vi "Appearance Page.vi"() -> ()   [LabVIEW 2017, in "2D Plot.lvclass"]
uses:
  <vilib>/Math Plots/2D Math Plots/2D Plot/2D Plot/2D Plot.lvclass
  <vilib>/Math Plots/2D Math Plots/2D Plot/2D Plot/Typedef/Graph General Property.ctl
  <vilib>/Math Plots/2D Math Plots/2D Plot/Action String/2DMathPlot Ctrl Act Queue.ctl
  <vilib>/Math Plots/2D Math Plots/2D Plot/Action String/2DMathPlot Ctrl Act Cluster.ctl
  <vilib>/Math Plots/2D Math Plots/2D Plot/Action String/2DMathPlot State Class.ctl
  <vilib>/Math Plots/2D Math Plots/2D Plot/2D Plot/Typedef/Dialog State.ctl
  <vilib>/Math Plots/2D Math Plots/2D Plot/2D Plot/Typedef/Temp Graph Property Action.ctl
  <vilib>/Math Plots/2D Math Plots/2D Plot/2D Plot/Typedef/Temp Graph State.ctl
panel:
  in  "Event Registration":refnum<event-registration>
  in  "Control Ref Queue":T1
  out "Graph General Out":T2
  in  "Graph General In":T2
  in  "Legend:Plots Shown":u32=1 caption="Plots shown" min=1
  in  "Autosize Legend":bool caption="Auto size to plot names"
  in  "Cursor Palette Visible":bool caption="Show cursor legend"
  in  "Legend:Visible":bool caption="Show plot legend"
  in  "Scale Legend:Visible":bool caption="Show scale legend"
  in  "Palette:Visible":bool caption="Show graph palette"
  in  "X Scrollbar Visible":bool caption="Show x scroll bar"
  in  "Height":u32 step=1
  in  "Width":u32 step=1
  in  "Enabled State":T3(radio)
  in  "Caption.Visible":bool caption="Caption"
  in  "Caption.Text":string caption="Caption Text"
  in  "Label.Text":string caption="Label Text"
  in  "Label.Visible":bool caption="Label"
  # "Caption"
  # "Label"
  # "Enabled State"
  # "Size"
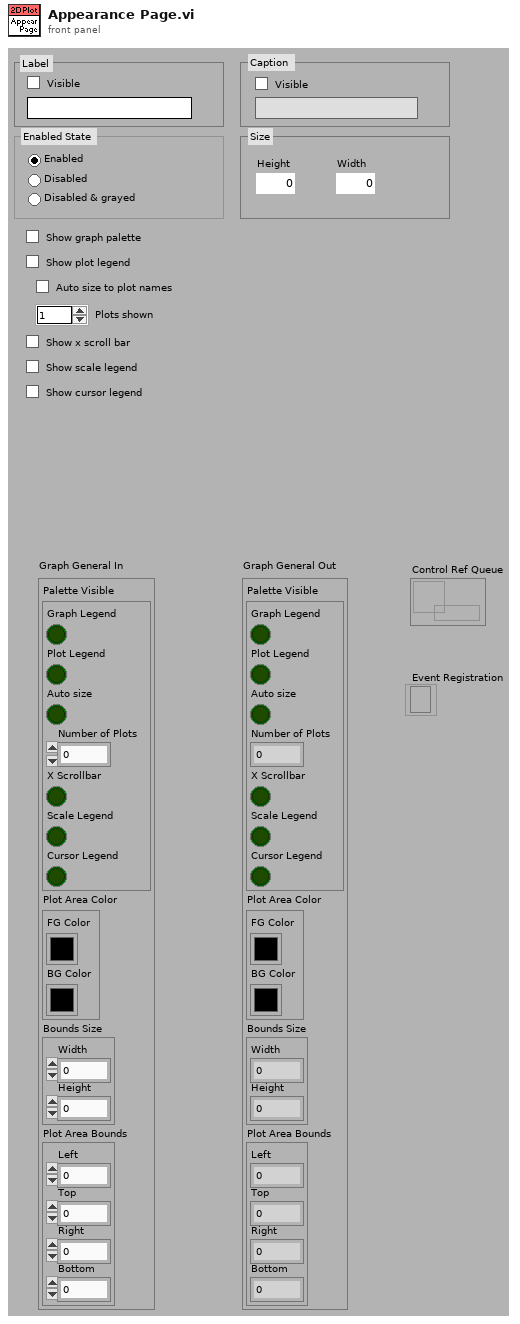
[diagram p1: front panel]
types:
  T1 = typedef "2DMathPlot Ctrl Act Queue.ctl" = refnum<queue>
  T2 = typedef "2D Plot.lvclass/Graph General Property.ctl" = cluster{"Palette Visible":cluster{"Graph Legend":bool, "Plot Legend":bool, "Auto size":bool, "Number of Plots":u32, "X Scrollbar":bool, "Scale Legend":bool, "Cursor Legend":bool}, "Plot Area Color":cluster{"FG Color":u32, "BG Color":u32}, "Bounds Size":cluster{"Width":u32, "Height":u32}, "Plot Area Bounds":cluster{"Left":i16, "Top":i16, "Right":i16, "Bottom":i16}}
  T3 = enum32{"Enabled", "Disabled", "Disabled & grayed", "Multiple Values"}
  T4 = typedef "2D Plot.lvclass/Dialog State.ctl" = enum16{"Initialize", "Read Property", "Write Property", "Idle", "Exit"}
  T5 = typedef "2DMathPlot Ctrl Act Cluster.ctl" = cluster{"Plot Area Ref":refnum<vi>, "Z Axis Ref":refnum<vi>, "Legend Ref":refnum<vi>, "XControl Ref":refnum<vi>, "Facade Ref":refnum<vi>, "Display State Change Class":T6}
  T6 = typedef "2DMathPlot State Class.ctl" = enum16{"Update All (Undo)", "Update General", "Update Appearance", "Update Format", "Update Scale", "Update Marker", "Update Cursor", "None"}
  T7 = typedef "2D Plot.lvclass/Temp Graph State.ctl" = enum16{"Create", "Update Graph", "Update Property Only", "Get Plot Name", "Get Axis Name", "Destory"}
  T8 = typedef "2D Plot.lvclass/Temp Graph Property Action.ctl" = enum16{"Appearance Property", "Format Property", "Plots Property", "Scales Property"}
  T9 = cluster{"Left":i16, "Top":i16, "Right":i16, "Bottom":i16}
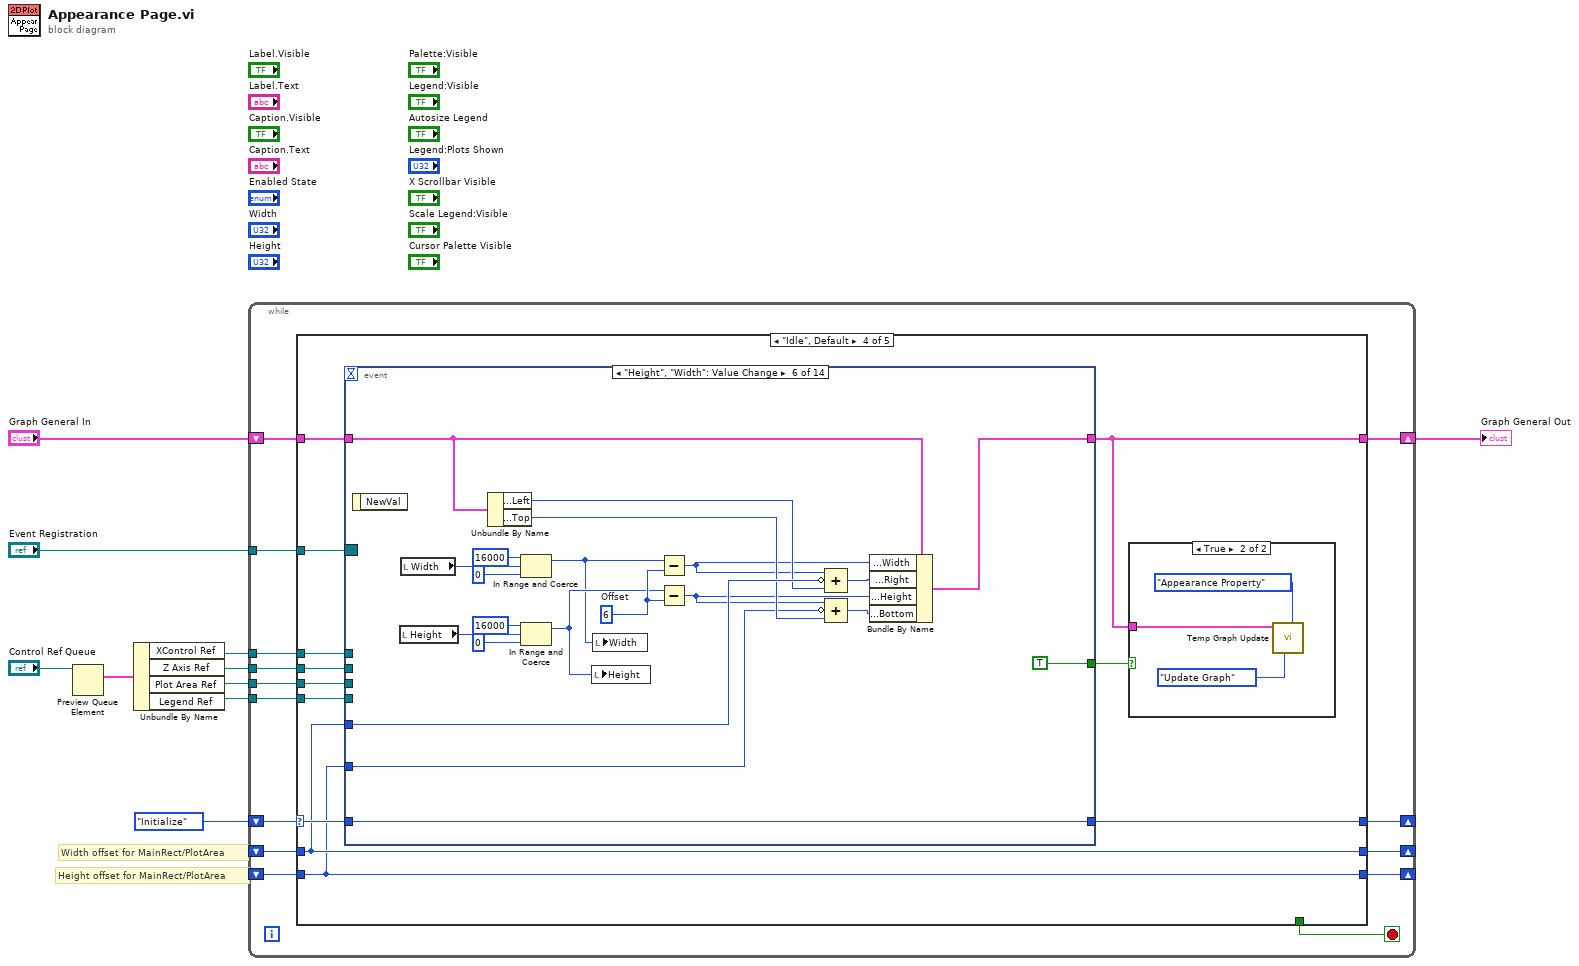
[diagram p0: block diagram]
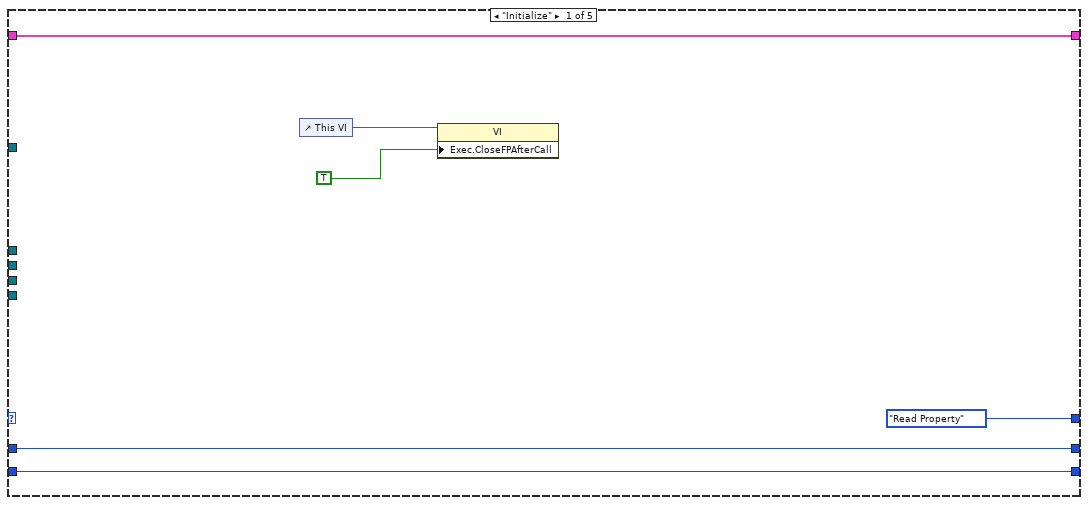
[diagram p2: hidden frame]
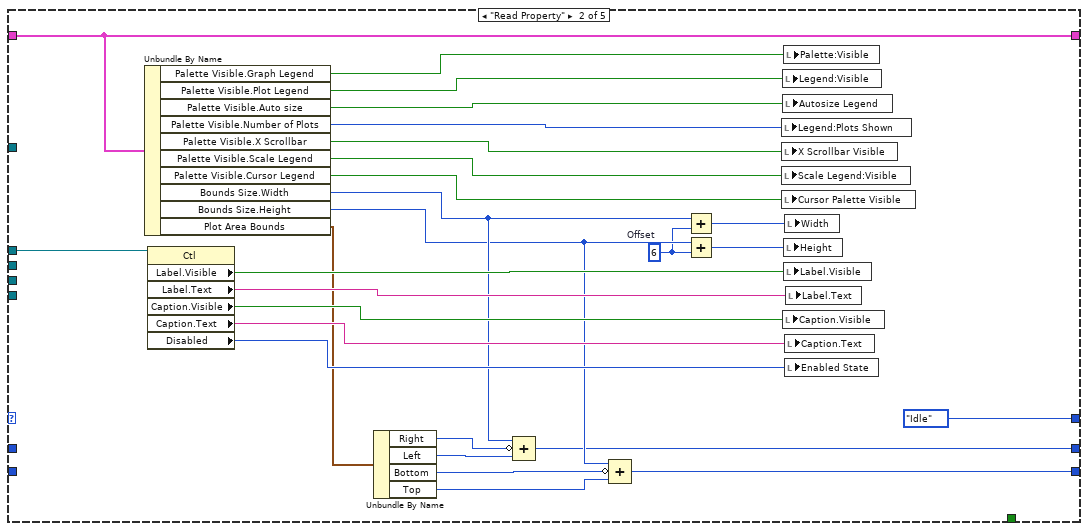
[diagram p3: hidden frame]
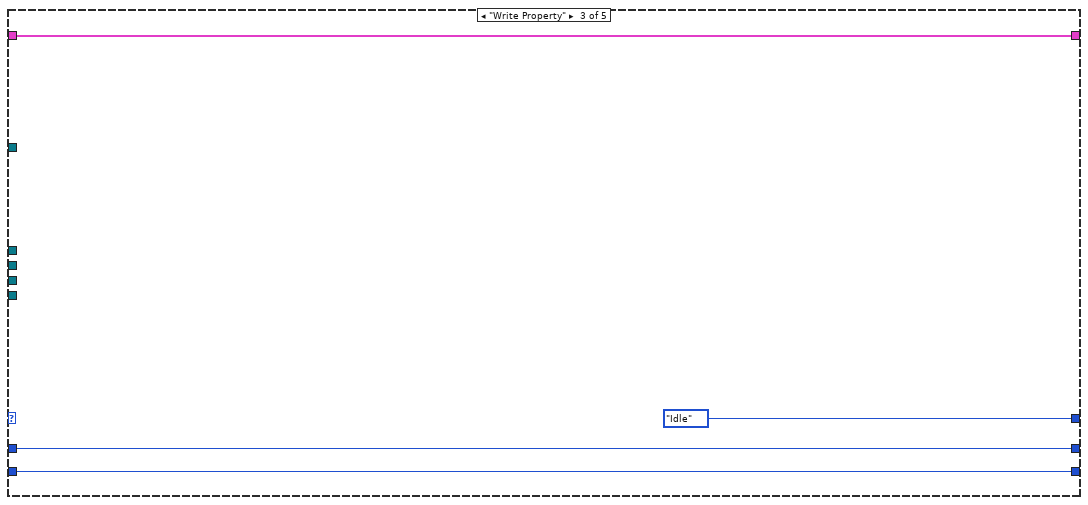
[diagram p4: hidden frame]
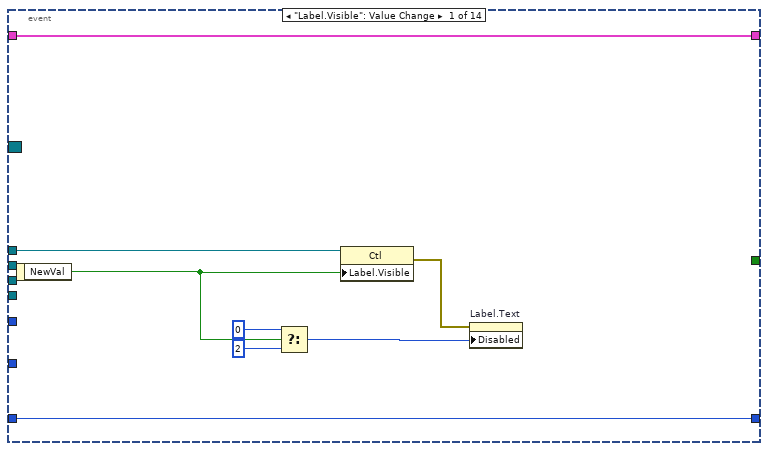
[diagram p6: hidden frame]
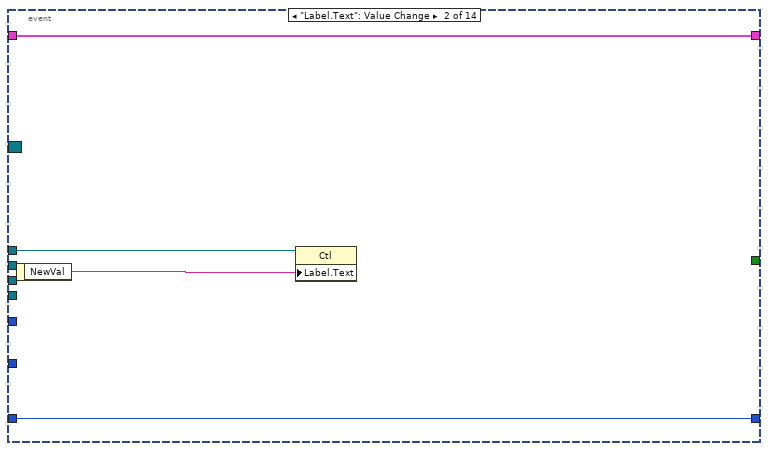
[diagram p7: hidden frame]
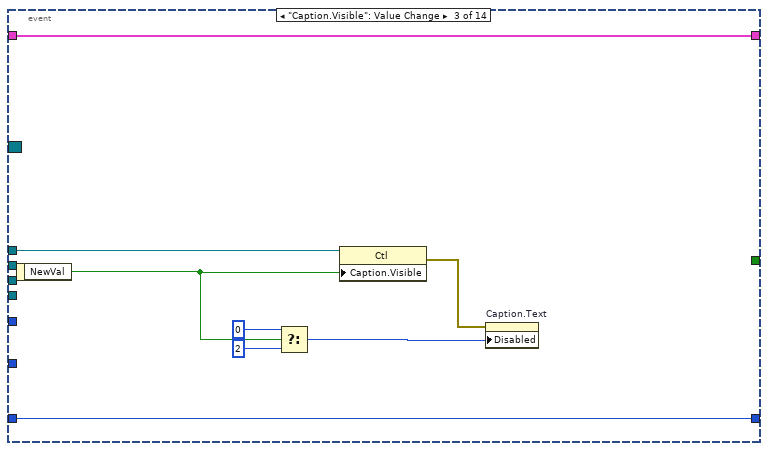
[diagram p8: hidden frame]
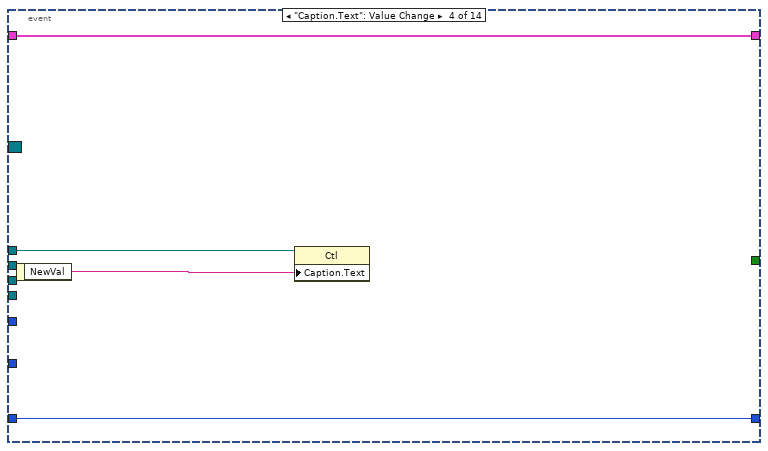
[diagram p9: hidden frame]
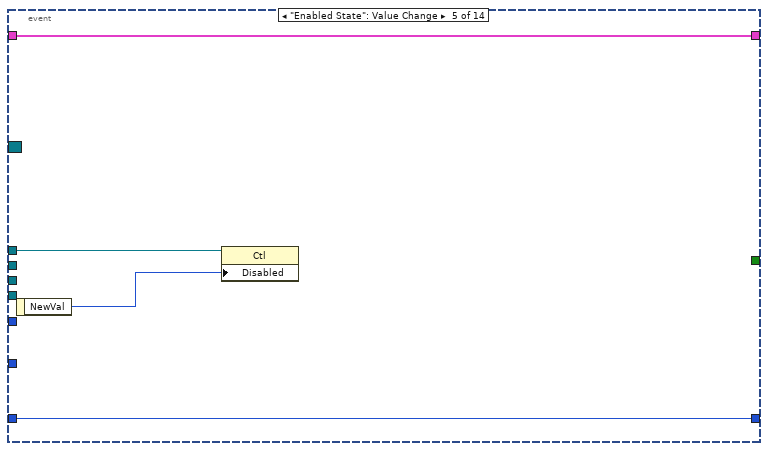
[diagram p10: hidden frame]
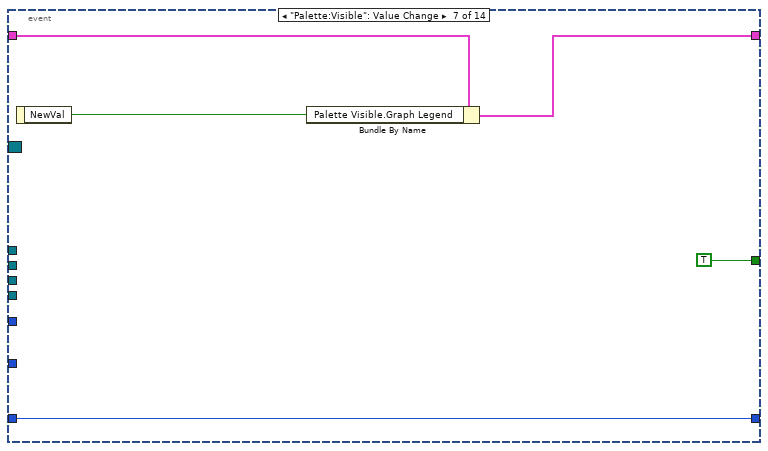
[diagram p11: hidden frame]
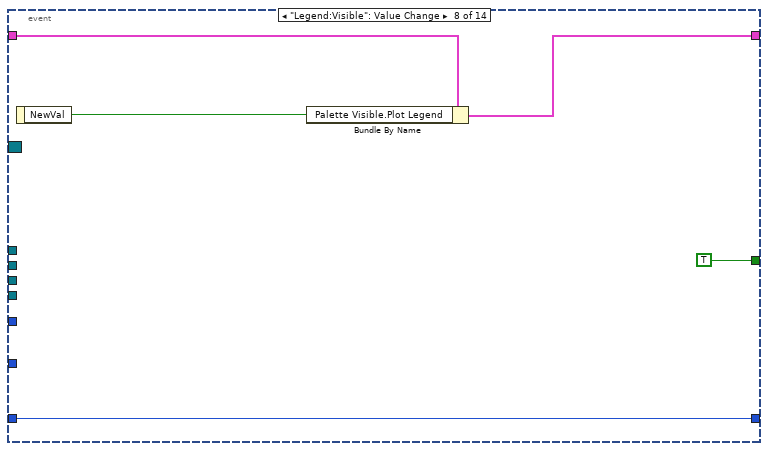
[diagram p12: hidden frame]
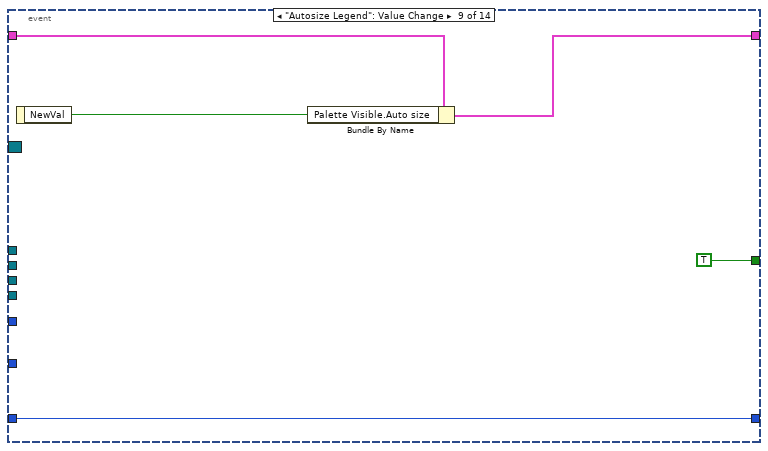
[diagram p13: hidden frame]
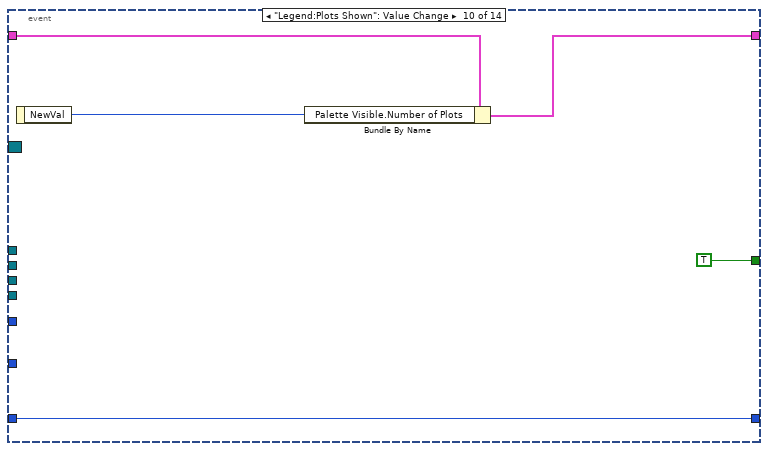
[diagram p14: hidden frame]
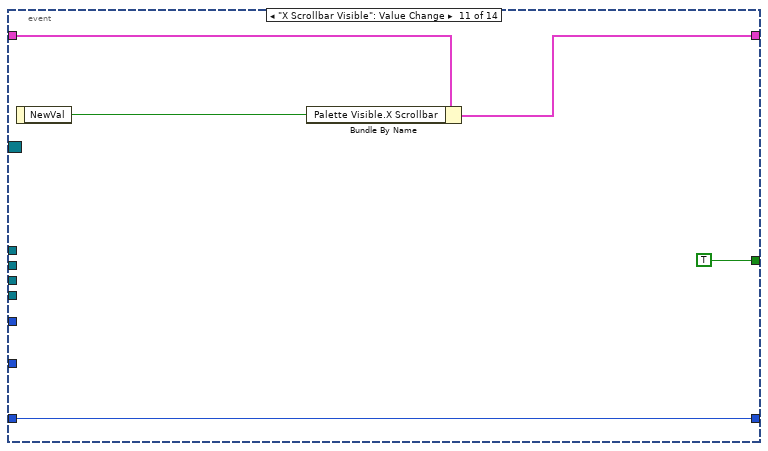
[diagram p15: hidden frame]
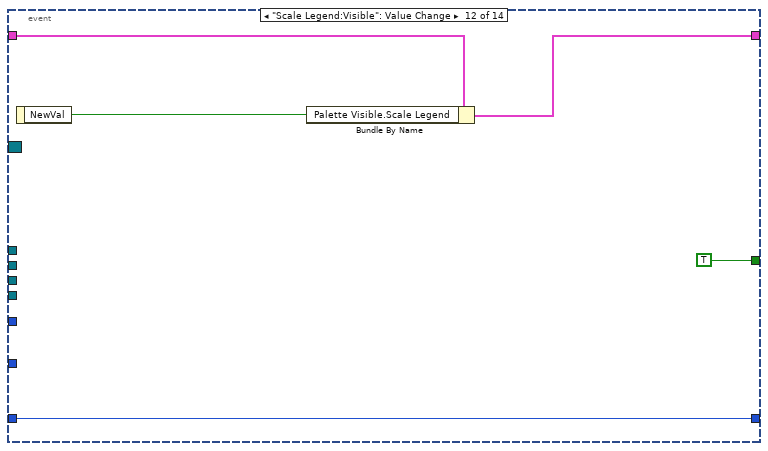
[diagram p16: hidden frame]
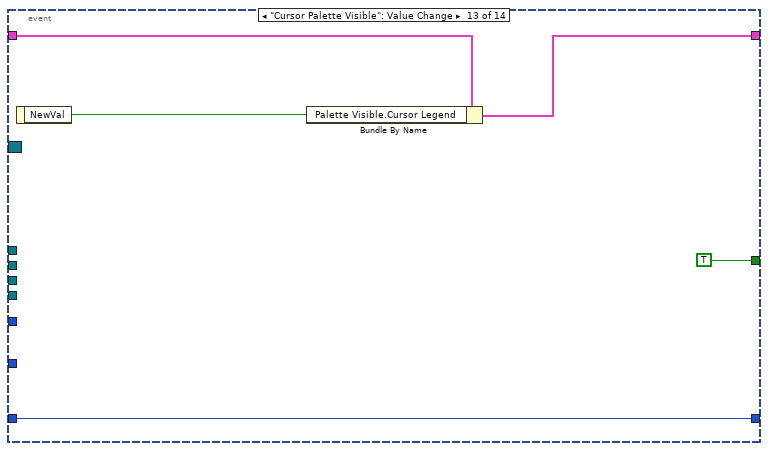
[diagram p17: hidden frame]
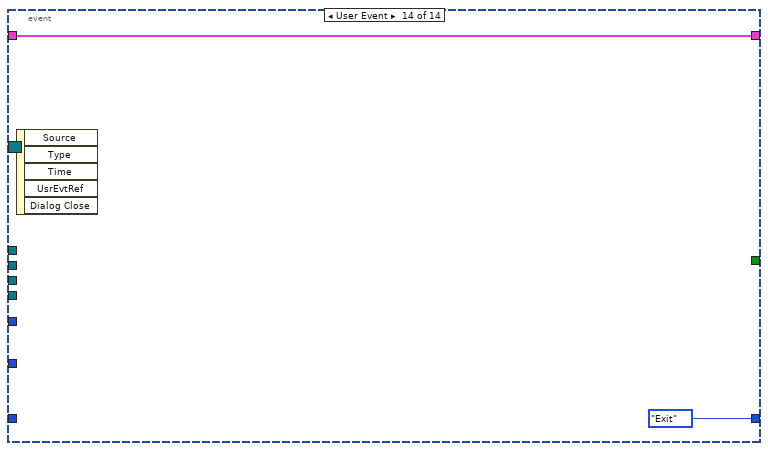
[diagram p18: hidden frame]
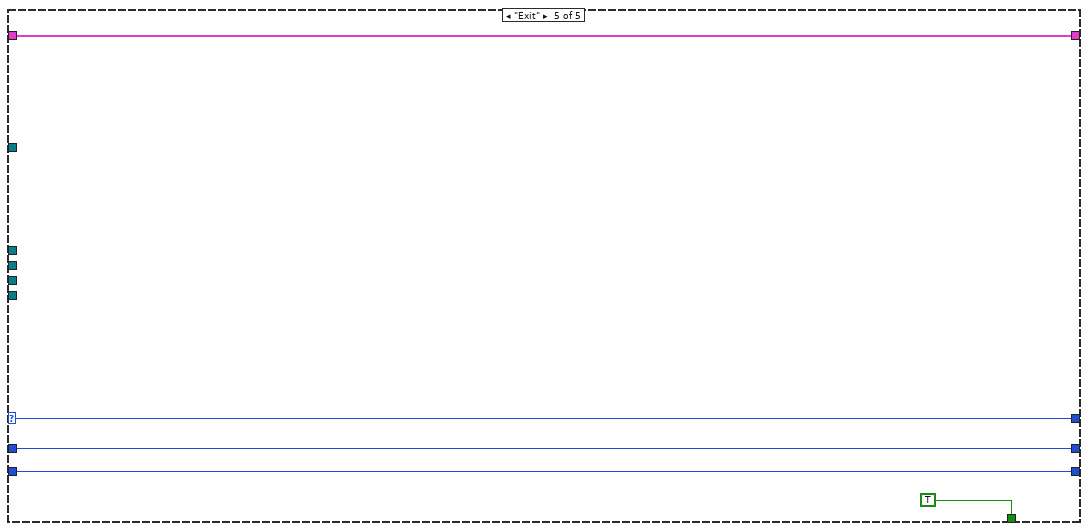
[diagram p19: hidden frame]
diagram:
  # "Height offset for MainRect/PlotArea"
  # "Width offset for MainRect/PlotArea"
  n1 = Preview Queue Element(queue="Control Ref Queue") -> (element=w2:T5)  [unwired: 1 in, 4 out]
  n2 = Unbundle By Name(w2) -> ("XControl Ref"=w6:refnum<vi>, "Z Axis Ref"=w5:refnum<vi>, "Plot Area Ref"=w4:refnum<vi>, "Legend Ref"=w1:refnum<vi>)
  n3 = while {
    shift-right: [w22] -> _
    shift-left: Dialog_State."Initialize" ("Enum") -> [w24]
    shift-right: [w21] -> w9
    shift-left: "Graph General In" -> [w20]
    tunnel: w6 -> [w19]
    tunnel: w5 -> [w18]
    tunnel: w4 -> [w17]
    tunnel: "Event Registration" -> [w16]
    shift-right: [w15] -> _
    shift-left: _ -> [w13]
    shift-right: [w14] -> _
    shift-left: _ -> [w12]
    tunnel: w1 -> [w11]
    stop <- w23 stop-if-true
    n4 = case shown="\"Idle\", Default" w24 {
      selector: w24 -> [_ _ _ w67 w166]
      tunnel: [_ _ _ _ TRUE] -> w23
      tunnel: [Dialog_State."Read Property" ("Enum") Dialog_State."Idle" ("Enum") Dialog_State."Idle" ("Enum") w68 w166] -> w22
      tunnel: [w27 w43 w60 w62 w165] -> w21
      tunnel: w20 -> [w27 w43 w60 w73 w165]
      tunnel: w19 -> [_ w49 _ w72 _]
      tunnel: w18 -> [_ _ _ w71 _]
      tunnel: w17 -> [_ _ _ w70 _]
      tunnel: w16 -> [_ _ _ w69 _]
      tunnel: [w26 w34 w59 w65 w164] -> w15
      tunnel: [w25 w35 w58 w64 w163] -> w14
      tunnel: w13 -> [w26 _ w59 w65 w164]
      tunnel: w12 -> [w25 _ w58 w64 w163]
      tunnel: w11 -> [_ _ _ w63 _]
      frame "Initialize" {
        n5 = control-ref of="This VI"() -> (w29:refnum<vi>)
        n6 = property class="VI"(reference=w29, "Exec.CloseFPAfterCall"=TRUE ("Execution:Close After Call")) -> ()  [unwired: 1 in, 2 out]
      }
      frame "Read Property" {
        w31 = u32 6  # Offset
        n7 = Unbundle By Name(w43) -> ("Palette Visible.Graph Legend"=w56:bool, "Palette Visible.Plot Legend"=w55:bool, "Palette Visible.Auto size"=w54:bool, "Palette Visible.Number of Plots"=w53:u32, "Palette Visible.X Scrollbar"=w52:bool, "Palette Visible.Scale Legend"=w51:bool, "Palette Visible.Cursor Legend"=w50:bool, "Bounds Size.Width"=w41:u32, "Bounds Size.Height"=w38:u32, "Plot Area Bounds"=w42:T9)
        n8 = property class="Ctl"(reference=w49) -> ("Label.Visible"=w48:bool, "Label.Text"=w47:string, "Caption.Visible"=w46:bool, "Caption.Text"=w45:string, "Disabled"=w44:u8)  [unwired: 1 in, 2 out]
        n9 = Unbundle By Name(w42) -> ("Right"=w40:i16, "Left"=w39:i16, "Bottom"=w37:i16, "Top"=w36:i16)
        n10 = Compound Arithmetic op=ADD(w41, invert w40, w39) -> (w34:u32)
        n11 = Compound Arithmetic op=ADD(w38, invert w37, w36) -> (w35:u32)
        n12 = Add(x=w41, y=w31) -> (x+y=w33:u32)
        n13 = Add(x=w38, y=w31) -> (x+y=w32:u32)
        n14 = local write "Legend:Plots Shown"(w53) -> ()
        n15 = local write "X Scrollbar Visible"(w52) -> ()
        n16 = local write "Scale Legend:Visible"(w51) -> ()
        n17 = local write "Cursor Palette Visible"(w50) -> ()
        n18 = local write "Legend:Visible"(w55) -> ()
        n19 = local write "Autosize Legend"(w54) -> ()
        n20 = local write "Caption.Visible"(w46) -> ()
        n21 = local write "Palette:Visible"(w56) -> ()
        n22 = local write "Height"(w32) -> ()
        n23 = local write "Label.Visible"(w48) -> ()
        n24 = local write "Width"(w33) -> ()
        n25 = local write "Caption.Text"(w45) -> ()
        n26 = local write "Enabled State"(w44) -> ()
        n27 = local write "Label.Text"(w47) -> ()
      }
      frame "Write Property" {
      }
      frame "Idle", Default {
        n28 = event shown="[5] \"Height\", \"Width\": Value Change" {
          selector: w69 -> [_ _ _ _ _ _ _ _ _ _ _ _ _ _]
          dyn-events: _ -> [_ _ _ _ _ _ _ _ _ _ _ _ _ _]
          timeout: _ -> [_ _ _ _ _ _ _ _ _ _ _ _ _ _]
          tunnel: w73 -> [w84 w86 w96 w98 w102 w122 w130 w135 w140 w145 w150 w155 w160 w162]
          tunnel: [w84 w86 w96 w98 w102 w124 w129 w134 w139 w144 w149 w154 w159 w162] -> w62
          tunnel: w72 -> [w83 w88 w95 w100 w104 _ _ _ _ _ _ _ _ _]
          tunnel: w71 -> [_ _ _ _ _ _ _ _ _ _ _ _ _ _]
          tunnel: w70 -> [_ _ _ _ _ _ _ _ _ _ _ _ _ _]
          tunnel: [w77 w85 w89 w97 w101 w125 w127 w132 w137 w142 w147 w152 w157 Dialog_State."Exit" ("Enum")] -> w68
          tunnel: w67 -> [w77 w85 w89 w97 w101 w125 w127 w132 w137 w142 w147 w152 w157 _]
          tunnel: [_ _ _ _ _ TRUE TRUE TRUE TRUE TRUE TRUE TRUE TRUE _] -> w66
          tunnel: w65 -> [_ _ _ _ _ w121 _ _ _ _ _ _ _ _]
          tunnel: w64 -> [_ _ _ _ _ w116 _ _ _ _ _ _ _ _]
          tunnel: w63 -> [_ _ _ _ _ _ _ _ _ _ _ _ _ _]
          event "Label.Visible": Value Change {
            n29 = event-data() -> ("NewVal"=w82:bool)  [unwired: 1 out]
            n30 = Select(t=u8 0 ("Disabled"), s=w82, f=u8 2 ("Disabled")) -> (s? t:f=w79:u8)
            n31 = property class="Ctl"(reference=w83, "Label.Visible"=w82) -> (error out=w78:errorcluster)  [unwired: 1 in, 1 out]
            n32 = property on="Label.Text" class="Str"(error in=w78, "Disabled"=w79) -> ()  [unwired: 1 in, 2 out]
          }
          event "Label.Text": Value Change {
            n33 = event-data() -> ("NewVal"=w87:string)  [unwired: 1 out]
            n34 = property class="Ctl"(reference=w88, "Label.Text"=w87) -> ()  [unwired: 1 in, 2 out]
          }
          event "Caption.Visible": Value Change {
            n35 = event-data() -> ("NewVal"=w94:bool)  [unwired: 1 out]
            n36 = Select(t=u8 0 ("Disabled"), s=w94, f=u8 2 ("Disabled")) -> (s? t:f=w91:u8)
            n37 = property class="Ctl"(reference=w95, "Caption.Visible"=w94) -> (error out=w90:errorcluster)  [unwired: 1 in, 1 out]
            n38 = property on="Caption.Text" class="Str"(error in=w90, "Disabled"=w91) -> ()  [unwired: 1 in, 2 out]
          }
          event "Caption.Text": Value Change {
            n39 = event-data() -> ("NewVal"=w99:string)  [unwired: 1 out]
            n40 = property class="Ctl"(reference=w100, "Caption.Text"=w99) -> ()  [unwired: 1 in, 2 out]
          }
          event "Enabled State": Value Change {
            n41 = event-data() -> ("NewVal"=w103:T3)  [unwired: 1 out]
            n42 = property class="Ctl"(reference=w104, "Disabled"=w103) -> ()  [unwired: 1 in, 2 out]
          }
          event "Height", "Width": Value Change {
            w115 = u32 6  # Offset
            n43 = event-data() -> ()  [unwired: 2 out]
            n44 = local read "Height"() -> (w110:u32)
            n45 = local read "Width"() -> (w107:u32)
            n46 = Unbundle By Name(w122) -> ("Plot Area Bounds.Left"=w120:i16, "Plot Area Bounds.Top"=w119:i16)
            n47 = In Range and Coerce(upper limit=u32 16000, x=w107, lower limit=u32 0) -> (coerced(x)=w105:u32)  [unwired: 1 out]
            n48 = In Range and Coerce(upper limit=u32 16000, x=w110, lower limit=u32 0) -> (coerced(x)=w106:u32)  [unwired: 1 out]
            n49 = local write "Height"(w106) -> ()
            n50 = local write "Width"(w105) -> ()
            n51 = Subtract(x=w105, y=w115) -> (x-y=w113:u32)
            n52 = Subtract(x=w106, y=w115) -> (x-y=w114:u32)
            n53 = Compound Arithmetic op=ADD(w113, invert w121, w120) -> (w117:u32)
            n54 = Compound Arithmetic op=ADD(w114, invert w116, w119) -> (w118:u32)
            n55 = Bundle By Name(cluster=w122, "Bounds Size.Width"=w113, "Plot Area Bounds.Right"=w117, "Bounds Size.Height"=w114, "Plot Area Bounds.Bottom"=w118) -> (w124:T2)
          }
          event "Palette:Visible": Value Change {
            n56 = event-data() -> ("NewVal"=w128:bool)  [unwired: 1 out]
            n57 = Bundle By Name(cluster=w130, "Palette Visible.Graph Legend"=w128) -> (w129:T2)
          }
          event "Legend:Visible": Value Change {
            n58 = event-data() -> ("NewVal"=w133:bool)  [unwired: 1 out]
            n59 = Bundle By Name(cluster=w135, "Palette Visible.Plot Legend"=w133) -> (w134:T2)
          }
          event "Autosize Legend": Value Change {
            n60 = event-data() -> ("NewVal"=w138:bool)  [unwired: 1 out]
            n61 = Bundle By Name(cluster=w140, "Palette Visible.Auto size"=w138) -> (w139:T2)
          }
          event "Legend:Plots Shown": Value Change {
            n62 = event-data() -> ("NewVal"=w143:u32)  [unwired: 1 out]
            n63 = Bundle By Name(cluster=w145, "Palette Visible.Number of Plots"=w143) -> (w144:T2)
          }
          event "X Scrollbar Visible": Value Change {
            n64 = event-data() -> ("NewVal"=w148:bool)  [unwired: 1 out]
            n65 = Bundle By Name(cluster=w150, "Palette Visible.X Scrollbar"=w148) -> (w149:T2)
          }
          event "Scale Legend:Visible": Value Change {
            n66 = event-data() -> ("NewVal"=w153:bool)  [unwired: 1 out]
            n67 = Bundle By Name(cluster=w155, "Palette Visible.Scale Legend"=w153) -> (w154:T2)
          }
          event "Cursor Palette Visible": Value Change {
            n68 = event-data() -> ("NewVal"=w158:bool)  [unwired: 1 out]
            n69 = Bundle By Name(cluster=w160, "Palette Visible.Cursor Legend"=w158) -> (w159:T2)
          }
          event User Event {
            n70 = event-data() -> ()  [unwired: 6 out]
          }
        }
        n71 = case shown="True" w66 {
          tunnel: w62 -> [_ w76]
          frame False {
          }
          frame True {
            n72 = call <vilib>:"Temp Graph Update.vi"("Property Name"=Temp_Graph_Property_Action."Appearance Property", "State"=Temp_Graph_State."Update Graph", "Property In"=w76) -> ()  [unwired: 2 in, 7 out]
          }
        }
      }
      frame "Exit" {
      }
    }
  }
  "Graph General Out" <- w9
